vi "Q15_transfer_1_Z.vi"(3 "Qn":dbl[](array[numeric]), 4 "x":dbl format="%#_13g") -> (1 "y":dbl)   [LabVIEW 2015]
panel:
  out "x*y 2":dbl[](array[numeric])
  out "xk chain":dbl[](array[numeric])
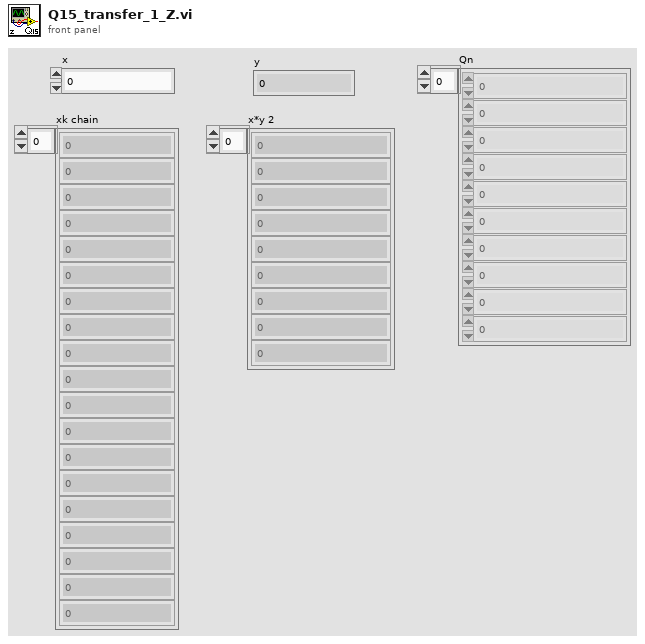
[diagram p1: front panel]
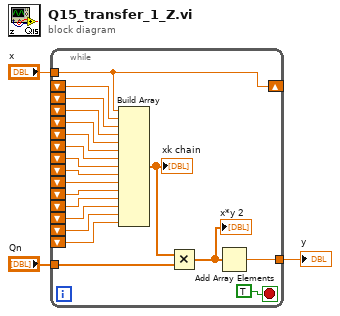
[diagram p0: block diagram]
diagram:
  n1 = while {
    tunnel: [w14] -> w3
    tunnel: "x" -> [w22]
    tunnel: "Qn" -> [w18]
    shift-right: [w22] -> _
    shift-left: _ -> [w21]
    shift-left: _ -> [w17]
    shift-left: _ -> [w16]
    shift-left: _ -> [w15]
    shift-left: _ -> [w13]
    shift-left: _ -> [w12]
    shift-left: _ -> [w11]
    shift-left: _ -> [w10]
    shift-left: _ -> [w9]
    shift-left: _ -> [w8]
    shift-left: _ -> [w7]
    shift-left: _ -> [w6]
    shift-left: _ -> [w5]
    shift-left: _ -> [w4]
    stop <- TRUE stop-if-true
    n2 = Build Array(w22, w21, w17, w16, w15, w13, w12, w11, w10, w9, w8, w7, w6, w5, w4) -> (w19:dbl[])
    "xk chain" <- w19
    n3 = Multiply(x=w19, y=w18) -> (x*y=w23:dbl[])
    "x*y 2" <- w23
    n4 = Add Array Elements(numeric array=w23) -> (sum=w14:dbl)
  }
  "y" <- w3
